vi "getCenter.vi"(6 "useControlBodyOnly":bool, 8 "error in (no error)":errorcluster, 11 "ref":refnum<vi>) -> (0 "error out":errorcluster, 2 "center":cluster{"horizontal":i32, "vertical":i32}, 3 "ref(dup)":refnum<vi>)   [LabVIEW 2023]
doc: "Returns the center point (X, Y) of the input control.\nThe calculation is based on the control bounds, optionally excluding captions and labels."
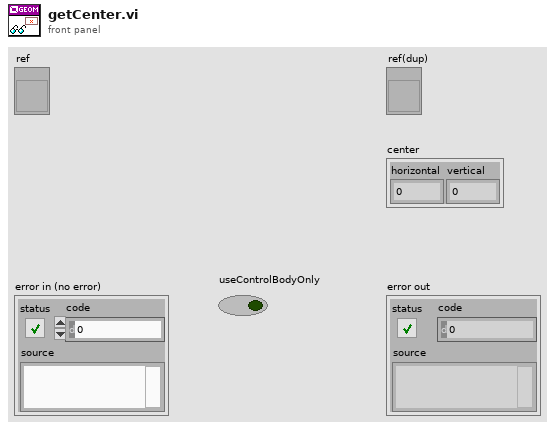
[diagram p1: front panel]
types:
  T1 = cluster{"left":i32, "top":i32, "right":i32, "bottom":i32}
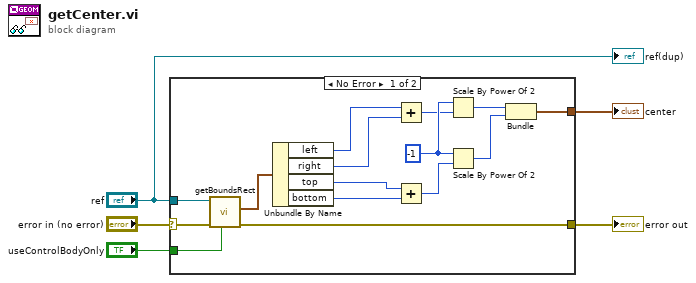
[diagram p0: block diagram]
diagram:
  n1 = case shown="No Error" "error in (no error)" {
    selector: "error in (no error)" -> [w20 w21]
    tunnel: [w17 _] -> w2
    tunnel: [w16 w21] -> w5
    tunnel: "ref" -> [w18 _]
    tunnel: "useControlBodyOnly" -> [w6 _]
    frame No Error {
      w13 = -1
      n2 = call "getBoundsRect.vi"("useControlBodyOnly"=w6, "error in (no error)"=w20, "ref"=w18) -> ("error out"=w16:errorcluster, "rect"=w19:T1)  [unwired: 6 in, 1 out]
      n3 = Unbundle By Name(w19) -> ("left"=w7:i32, "right"=w8:i32, "top"=w9:i32, "bottom"=w10:i32)
      n4 = Add(x=w7, y=w8) -> (x+y=w12:i32)
      n5 = Add(x=w9, y=w10) -> (x+y=w11:i32)
      n6 = Scale By Power Of 2(n=w13, x=w12) -> (x*2^n=w14:i32)
      n7 = Scale By Power Of 2(n=w13, x=w11) -> (x*2^n=w15:i32)
      n8 = Bundle(w14, w15) -> (w17:cluster{i32, i32})  [unwired: 1 in]
    }
    frame Error {
    }
  }
  "error out" <- w5
  "center" <- w2
  "ref(dup)" <- "ref"
